vi "AIT 664 - Add Tx Message Port.vi"(0 "Item Ref in":T4 format="%.0x", 5 "Tx Message Port":T1, 11 "error in (no error)":errorcluster) -> (15 "error out":errorcluster)   [LabVIEW 2013, in "AIT 664 Custom Device.lvlib"]
doc: "Add Tx Message Port"
uses:
  AIT 664 Custom Device.lvlib
  <vilib>/NI Veristand/Custom Device API/Custom Device Item Ref.ctl
  Controls/664 - XML Tx Message Port.ctl
  Controls/664 - Sampling Type.ctl
  Controls/664 -Param.ctl
  <vilib>/NI Veristand/Custom Device API/Custom Device Channel Type.ctl
  <vilib>/NI Veristand/Custom Device API/Custom Device Channel.ctl
  Controls and Global/Global.vi
  <vilib>/NI Veristand/Custom Device API/Set Item Property (U32).vi
  <vilib>/NI Veristand/Custom Device API/Set Item Property (Variant).vi
  <vilib>/NI Veristand/Custom Device API/Set Item Property (String).vi
  <vilib>/NI Veristand/Custom Device API/Set Item Property (Boolean).vi
  <vilib>/NI Veristand/Custom Device API/Custom Device API.lvlib
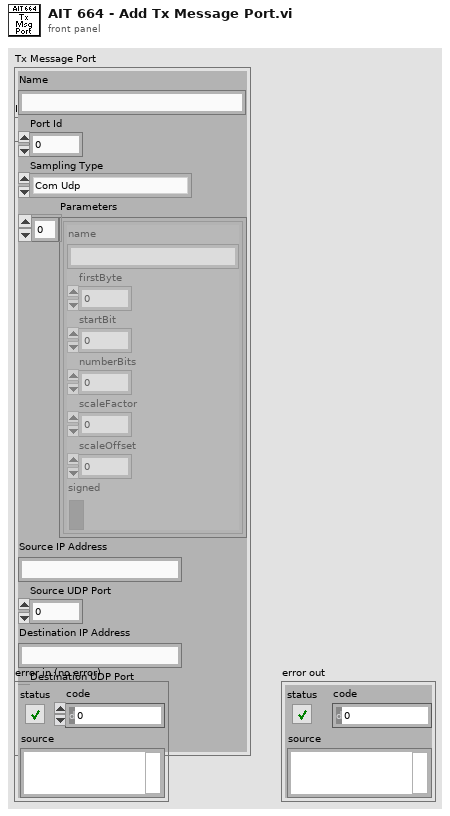
[diagram p1: front panel]
types:
  T1 = typedef "AIT 664 Custom Device.lvlib/664 - XML Tx Message Port.ctl" = cluster{"Name":string, "Port Id":u32, "Sampling Type":T2, "Parameters":T3[], "Source IP Address":string, "Source UDP Port":u32, "Destination IP Address":string, "Destination UDP Port":u32, "Tx Rate (ms)":u32}
  T2 = typedef "AIT 664 Custom Device.lvlib/664 - Sampling Type.ctl" = enum16{"Com Udp", "Com Udp Queuing", "Sap Udp", "Sap Ip", "Sap Mac", "Unknown"}
  T3 = typedef "AIT 664 Custom Device.lvlib/664 -Param.ctl" = cluster{"name":string, "firstByte":i32, "startBit":i32, "numberBits":i32, "scaleFactor":dbl, "scaleOffset":dbl, "signed":bool}
  T4 = typedef "Custom Device API.lvlib/Custom Device Item Ref.ctl" = u64
  T5 = typedef "Custom Device API.lvlib/Custom Device Channel Type.ctl" = enum16{"Input", "Output"}
  T6 = typedef "Custom Device API.lvlib/Custom Device Channel.ctl" = cluster{"Type":T5, "Units":string, "Default Value":dbl, "Faultable":bool, "Scalable":bool}
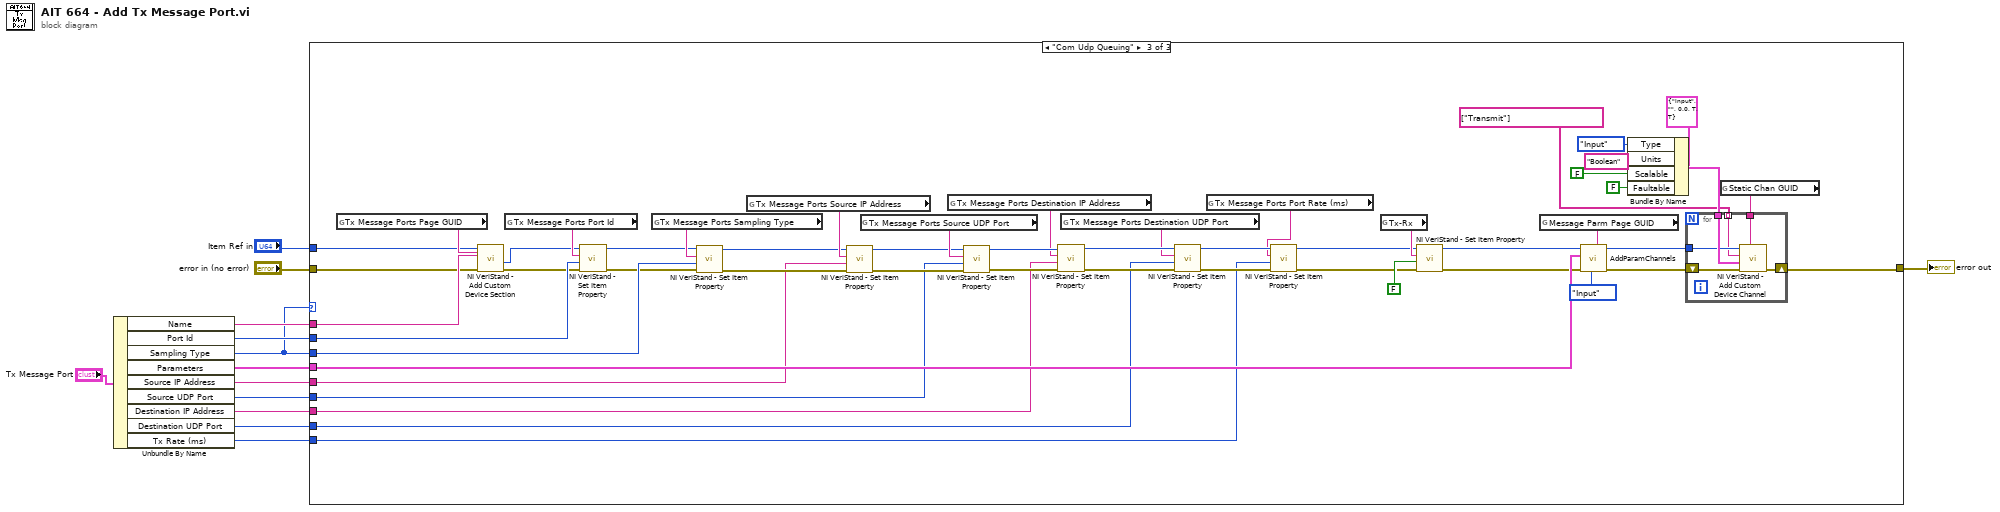
[diagram p0: block diagram]
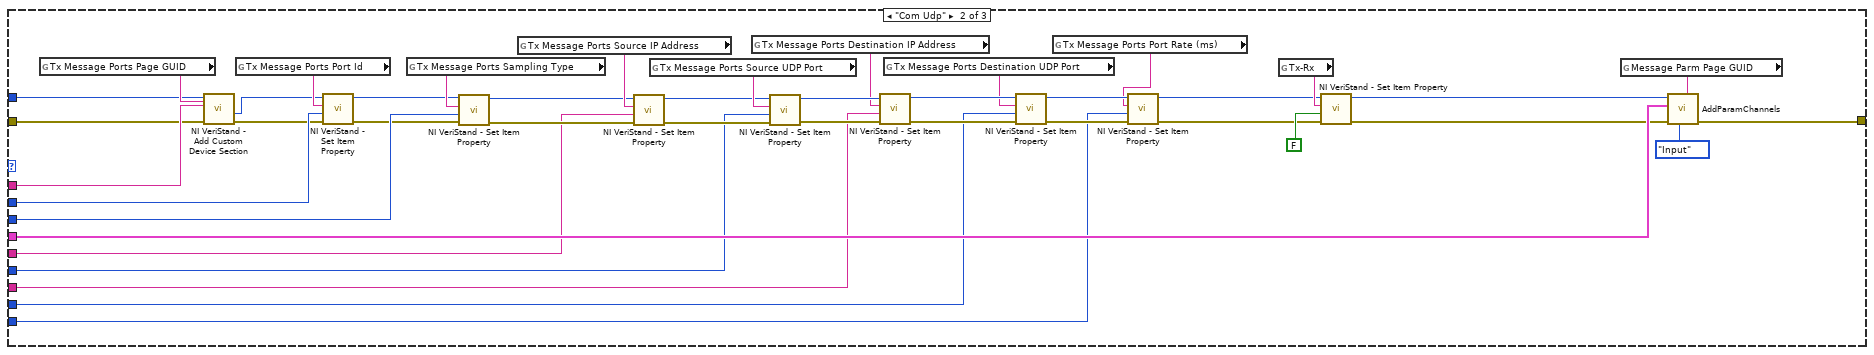
[diagram p3: hidden frame]
diagram:
  n1 = Unbundle By Name("Tx Message Port") -> ("Name"=w12:string, "Port Id"=w13:u32, "Sampling Type"=w9:T2, "Parameters"=w10:T3[], "Source IP Address"=w6:string, "Source UDP Port"=w5:u32, "Destination IP Address"=w4:string, "Destination UDP Port"=w3:u32, "Tx Rate (ms)"=w2:u32)
  n2 = case shown="\"Com Udp Queuing\"" w9 {
    tunnel: w9 -> [_ w55 w107]
    tunnel: w13 -> [_ w51 w103]
    tunnel: w12 -> [_ w47 w99]
    tunnel: w10 -> [_ w44 w96]
    tunnel: "error in (no error)" -> [w14 w43 w95]
    tunnel: [w14 w42 w73] -> w7
    tunnel: w6 -> [_ w30 w83]
    tunnel: w5 -> [_ w29 w82]
    tunnel: w4 -> [_ w28 w81]
    tunnel: w3 -> [_ w27 w80]
    tunnel: w2 -> [_ w22 w75]
    tunnel: "Item Ref in" -> [_ w21 w66]
    frame "Sap Udp".."Unknown", Default {
    }
    frame "Com Udp" {
      n3 = global read "Global.vi" "Tx Message Ports Page GUID"() -> (w48:string)
      n4 = call <vilib>:"NI VeriStand - Add Custom Device Section.vi"("GUID (Default Section)"=w48, "error in (no error)"=w43, "Section Name"=w47, "Parent Ref in"=w21) -> ("error out"=w49:errorcluster, "Section Ptr"=w50:T4)  [unwired: 4 in, 2 out]
      n5 = global read "Global.vi" "Tx Message Ports Port Id"() -> (w52:string)
      n6 = call-poly <vilib>:"NI VeriStand - Set Item Property.vi"("error in (no error)"=w49, "Value"=w51, "Property Name"=w52, "Item Ref in"=w50) -> ("error out"=w53:errorcluster, "Item Ref out"=w54:T4)  [unwired: 5 in, 1 out]
      n7 = global read "Global.vi" "Tx Message Ports Sampling Type"() -> (w56:string)
      n8 = call-poly <vilib>:"NI VeriStand - Set Item Property.vi"("error in (no error)"=w53, "Value"=w55, "Property Name"=w56, "Item Ref in"=w54) -> ("error out"=w32:errorcluster, "Item Ref out"=w31:T4)  [unwired: 5 in, 1 out]
      n9 = global read "Global.vi" "Tx Message Ports Source IP Address"() -> (w33:string)
      n10 = call-poly <vilib>:"NI VeriStand - Set Item Property.vi"("error in (no error)"=w32, "Value"=w30, "Property Name"=w33, "Item Ref in"=w31) -> ("error out"=w34:errorcluster, "Item Ref out"=w35:T4)  [unwired: 5 in, 1 out]
      n11 = global read "Global.vi" "Tx Message Ports Source UDP Port"() -> (w36:string)
      n12 = global read "Global.vi" "Tx Message Ports Destination IP Address"() -> (w39:string)
      n13 = call-poly <vilib>:"NI VeriStand - Set Item Property.vi"("error in (no error)"=w34, "Value"=w29, "Property Name"=w36, "Item Ref in"=w35) -> ("error out"=w40:errorcluster, "Item Ref out"=w41:T4)  [unwired: 5 in, 1 out]
      n14 = call-poly <vilib>:"NI VeriStand - Set Item Property.vi"("error in (no error)"=w40, "Value"=w28, "Property Name"=w39, "Item Ref in"=w41) -> ("error out"=w38:errorcluster, "Item Ref out"=w37:T4)  [unwired: 5 in, 1 out]
      n15 = global read "Global.vi" "Tx Message Ports Destination UDP Port"() -> (w26:string)
      n16 = call-poly <vilib>:"NI VeriStand - Set Item Property.vi"("error in (no error)"=w38, "Value"=w27, "Property Name"=w26, "Item Ref in"=w37) -> ("error out"=w25:errorcluster, "Item Ref out"=w24:T4)  [unwired: 5 in, 1 out]
      n17 = global read "Global.vi" "Tx Message Ports Port Rate (ms)"() -> (w23:string)
      n18 = call-poly <vilib>:"NI VeriStand - Set Item Property.vi"("error in (no error)"=w25, "Value"=w22, "Property Name"=w23, "Item Ref in"=w24) -> ("error out"=w18:errorcluster, "Item Ref out"=w16:T4)  [unwired: 5 in, 1 out]
      n19 = global read "Global.vi" "Tx-Rx"() -> (w19:string)
      n20 = call-poly <vilib>:"NI VeriStand - Set Item Property.vi"("error in (no error)"=w18, "Value"=FALSE, "Property Name"=w19, "Item Ref in"=w16) -> ("error out"=w17:errorcluster, "Item Ref out"=w15:T4)  [unwired: 5 in, 1 out]
      n21 = global read "Global.vi" "Message Parm Page GUID"() -> (w45:string)
      n22 = call "AddParamChannels.vi"("Parm Page GUID"=w45, "Type"=Custom_Device_Channel_Type."Input", "error in"=w17, "Parameters to add"=w44, "Node Ref In"=w15) -> ("error out"=w42:errorcluster)  [unwired: 5 in, 1 out]
    }
    frame "Com Udp Queuing" {
      n23 = global read "Global.vi" "Tx Message Ports Page GUID"() -> (w100:string)
      n24 = call <vilib>:"NI VeriStand - Add Custom Device Section.vi"("GUID (Default Section)"=w100, "error in (no error)"=w95, "Section Name"=w99, "Parent Ref in"=w66) -> ("error out"=w101:errorcluster, "Section Ptr"=w102:T4)  [unwired: 4 in, 2 out]
      n25 = global read "Global.vi" "Tx Message Ports Port Id"() -> (w104:string)
      n26 = call-poly <vilib>:"NI VeriStand - Set Item Property.vi"("error in (no error)"=w101, "Value"=w103, "Property Name"=w104, "Item Ref in"=w102) -> ("error out"=w105:errorcluster, "Item Ref out"=w106:T4)  [unwired: 5 in, 1 out]
      n27 = global read "Global.vi" "Tx Message Ports Sampling Type"() -> (w108:string)
      n28 = call-poly <vilib>:"NI VeriStand - Set Item Property.vi"("error in (no error)"=w105, "Value"=w107, "Property Name"=w108, "Item Ref in"=w106) -> ("error out"=w85:errorcluster, "Item Ref out"=w84:T4)  [unwired: 5 in, 1 out]
      n29 = global read "Global.vi" "Tx Message Ports Source IP Address"() -> (w86:string)
      n30 = call-poly <vilib>:"NI VeriStand - Set Item Property.vi"("error in (no error)"=w85, "Value"=w83, "Property Name"=w86, "Item Ref in"=w84) -> ("error out"=w87:errorcluster, "Item Ref out"=w88:T4)  [unwired: 5 in, 1 out]
      n31 = global read "Global.vi" "Tx Message Ports Source UDP Port"() -> (w89:string)
      n32 = global read "Global.vi" "Tx Message Ports Destination IP Address"() -> (w92:string)
      n33 = call-poly <vilib>:"NI VeriStand - Set Item Property.vi"("error in (no error)"=w87, "Value"=w82, "Property Name"=w89, "Item Ref in"=w88) -> ("error out"=w93:errorcluster, "Item Ref out"=w94:T4)  [unwired: 5 in, 1 out]
      n34 = call-poly <vilib>:"NI VeriStand - Set Item Property.vi"("error in (no error)"=w93, "Value"=w81, "Property Name"=w92, "Item Ref in"=w94) -> ("error out"=w91:errorcluster, "Item Ref out"=w90:T4)  [unwired: 5 in, 1 out]
      n35 = global read "Global.vi" "Tx Message Ports Destination UDP Port"() -> (w79:string)
      n36 = call-poly <vilib>:"NI VeriStand - Set Item Property.vi"("error in (no error)"=w91, "Value"=w80, "Property Name"=w79, "Item Ref in"=w90) -> ("error out"=w78:errorcluster, "Item Ref out"=w77:T4)  [unwired: 5 in, 1 out]
      n37 = global read "Global.vi" "Tx Message Ports Port Rate (ms)"() -> (w76:string)
      n38 = call-poly <vilib>:"NI VeriStand - Set Item Property.vi"("error in (no error)"=w78, "Value"=w75, "Property Name"=w76, "Item Ref in"=w77) -> ("error out"=w60:errorcluster, "Item Ref out"=w58:T4)  [unwired: 5 in, 1 out]
      n39 = global read "Global.vi" "Tx-Rx"() -> (w61:string)
      n40 = call-poly <vilib>:"NI VeriStand - Set Item Property.vi"("error in (no error)"=w60, "Value"=FALSE, "Property Name"=w61, "Item Ref in"=w58) -> ("error out"=w59:errorcluster, "Item Ref out"=w57:T4)  [unwired: 5 in, 1 out]
      n41 = global read "Global.vi" "Message Parm Page GUID"() -> (w97:string)
      n42 = call "AddParamChannels.vi"("Parm Page GUID"=w97, "Type"=Custom_Device_Channel_Type."Input", "error in"=w59, "Parameters to add"=w96, "Node Ref In"=w57) -> ("error out"=w74:errorcluster, "Node Ref Out"=w72:T4)  [unwired: 5 in]
      n43 = Bundle By Name(cluster=T6 {"Type"=enum."Input", "Units"="", "Default Value"=0.0, "Faultable"=TRUE, "Scalable"=TRUE} ("Channel"), "Type"=Custom_Device_Channel_Type."Input", "Units"="Boolean", "Scalable"=FALSE, "Faultable"=FALSE) -> (w69:T6)
      n44 = global read "Global.vi" "Static Chan GUID"() -> (w71:string)
      n45 = for {
        tunnel: w69 -> [w114]
        tunnel: w71 -> [w113]
        tunnel: w72 -> [w112]
        tunnel: string[] ["Transmit"] -> [w111] mode=indexing
        shift-right: [w110] -> w73
        shift-left: w74 -> [w109]
        n46 = call <vilib>:"NI VeriStand - Add Custom Device Channel.vi"("GUID (Default Channel)"=w113, "error in (no error)"=w109, "Channel"=w114, "Channel Name"=w111, "Parent Ref in"=w112) -> ("error out"=w110:errorcluster)  [unwired: 3 in, 3 out]
      }
    }
  }
  "error out" <- w7
